vi "ArrayToImage.vi"(6 "Image Pixels (Float)":sgl[][](array[numeric]) format="%.2f", 7 "Image Pixels (U16)":u16[][](array[numeric]), 8 "error in (no error)":errorcluster, 9 "Image Pixels (I16)":i16[][](array[numeric]), 10 "Image Pixels (U8)":u8[][](array[numeric]), 11 "Image":T1) -> (0 "error out":errorcluster, 3 "Image Out":T1)   [LabVIEW 2011]
doc: "Creates an image from a 2D array."
uses:
  <vilib>/vision/Image Controls.llb/IMAQ Image.ctl
  nivision.dll
panel:
  # "Y axis\nX axis"
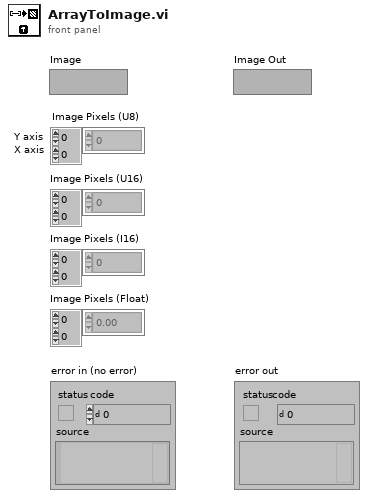
[diagram p1: front panel]
types:
  T1 = typedef "IMAQ Image.ctl" = refnum<image>
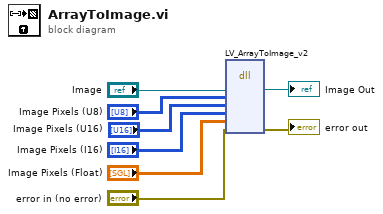
[diagram p0: block diagram]
diagram:
  n1 = dll-call lib="nivision.*" fn="LV_ArrayToImage_v2"("Image"="Image", "u8Handle"="Image Pixels (U8)", "u16Handle"="Image Pixels (U16)", "i16Handle"="Image Pixels (I16)", "sglHandle"="Image Pixels (Float)", "error in (no error)"="error in (no error)") -> ("Image"=→"Image Out":T1, "error in (no error)"=→"error out":errorcluster)  [unwired: 7 in, 3 out]
